vi "ROI entry-Init Cool Down ctrls.vi"(8 "error in (no error)":errorcluster) -> (0 "error out":errorcluster)   [LabVIEW 2013]
uses:
  ROI Entry screen/Globals/gl_ROI Entry UI globals.vi
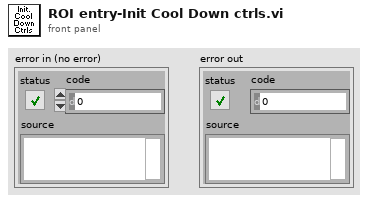
[diagram p1: front panel]
types:
  T1 = enum8{"Enabled", "Disabled", "Disabled and Grayed Out"}
  T2 = typedef "ROI entry screen ctrl refs cluster.ctl" = cluster{"Done button":refnum<vi>, "Imaging button":refnum<vi>, "Acquisition button":refnum<vi>, "POI dwell time (us)":refnum<vi>, "Scan dwell time per pixel (us)":refnum<vi>, "# of planes":refnum<vi>, "Zoom":refnum<vi>, "Equal size":refnum<vi>, "Channel":refnum<vi>, "Image Display":refnum<vi>, "Z-Plane Selector":refnum<vi>, "Number of lines left":refnum<vi>, "Z-stack folder path":refnum<vi>, "POI Density":refnum<vi>, "Arb Plane Entry":refnum<vi>, "Whole plane":refnum<vi>, "Clear Last":refnum<vi>, "Clear All":refnum<vi>, "Trial Length (sec)":refnum<vi>, "Palette Type":refnum<vi>, "Intensity slider":refnum<vi>, "# POI":refnum<vi>, "Max Z Proj":refnum<vi>, "Zplane ind":refnum<vi>, "Wavelength (nm)":refnum<vi>, "Number of Trials":refnum<vi>, "Funct stim.trig.enable":refnum<vi>, "Funct stim.trig.delay (s)":refnum<vi>, "Line Mode":refnum<vi>, "Step size (µm)":refnum<vi>, "ROI move mode":refnum<vi>, "Cool-down time (s)":refnum<vi>, "Enable cool-down time":refnum<vi>, "Motor Z ind. (um)":refnum<vi>, "AOL Z ind. (um)":refnum<vi>}
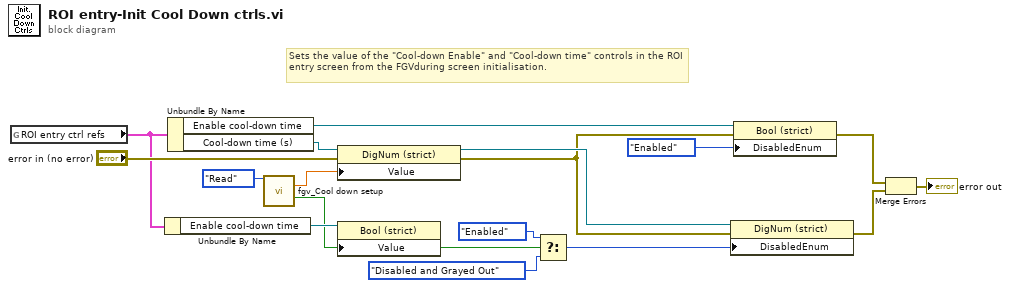
[diagram p0: block diagram]
diagram:
  # "Sets the value of the \"Cool-down Enable\" and \"Cool-down time\" controls in the ROI entry screen from the FGVduring screen initialisation."
  n1 = global read "gl_ROI Entry UI globals.vi" "ROI entry ctrl refs"() -> (w16:T2)
  n2 = Unbundle By Name(w16) -> ("Enable cool-down time"=w7:refnum<vi>)
  n3 = Unbundle By Name(w16) -> ("Enable cool-down time"=w13:refnum<vi>, "Cool-down time (s)"=w6:refnum<vi>)
  n4 = call "fgv_Cool down setup.vi"("Function"=enum16{"Intialize", "Write", "Read", "Clear"}."Read") -> ("Cool-down time (s)"=w2:dbl, "Enable cool-down time"=w1:bool)  [unwired: 12 in, 1 out]
  n5 = property on="Property Node" class="DigNum (strict)"(reference=w6, error in="error in (no error)", "Value"=w2) -> (reference out=w14:refnum<vi>, error out=w11:errorcluster)
  n6 = property on="Property Node" class="Bool (strict)"(reference=w7, "Value"=w1) -> ()  [unwired: 1 in, 2 out]
  n7 = Select(t=T1."Enabled" ("Disabled"), s=w1, f=T1."Disabled and Grayed Out" ("Disabled")) -> (s? t:f=w15:T1)
  n8 = property on="Property Node" class="DigNum (strict)"(reference=w14, error in=w11, "DisabledEnum"=w15) -> (error out=w10:errorcluster)  [unwired: 1 out]
  n9 = property on="Property Node" class="Bool (strict)"(reference=w13, error in=w11, "DisabledEnum"=T1."Enabled" ("Disabled")) -> (error out=w9:errorcluster)  [unwired: 1 out]
  n10 = Merge Errors(w9, w10) -> (→"error out":errorcluster)
